vi "Open Front Panel.vi"(6 "Custom Size":cluster{"Height":i16, "Width":i16}, 8 "error in (no error)":errorcluster, 9 "Custom Position":cluster{"Top":i16, "Left":i16}, 10 "Position":T1, 11 "MediatorBusMonitor in":refnum<class "MediatorBusMonitor.lvclass">) -> (0 "error out":errorcluster, 3 "MediatorBusMonitor out":refnum<class "MediatorBusMonitor.lvclass">)   [LabVIEW 2017, in "Mediator.lvlib" / "MediatorBusMonitor.lvclass"]
doc: "<License>\nCopyright © 2017 Composed Systems, LLC | All rights reserved\nwww.composed.io\n\nAuthor: Ethan Stern <ethan.stern@composed.io>\n\nThis software is provided \"AS IS\" WITHOUT WARRANTIES, either express or implied, AND IS FOR EDUCATIONAL PURPOSES ONLY.\n</License>"
uses:
  MediatorBusMonitor.lvclass
  IViewable/IViewable/View Position Enum.ctl
  MediatorBusMonitor.lvclass/MediatorBusMonitor.ctl
  IMediator/IMediatorBusMonitor/MediatorBusMonitor/IMediatorBusMonitor.lvclass
  IViewable/IViewable/IViewable.lvclass
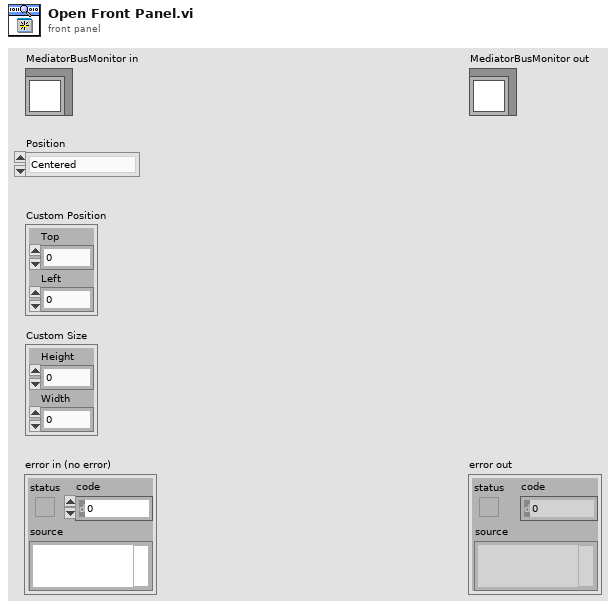
[diagram p1: front panel]
types:
  T1 = typedef "IViewable.lvlib/IViewable.lvclass/View Position Enum.ctl" = enum16{"Centered", "Maximized", "Minimized", "Custom", "Unchanged"}
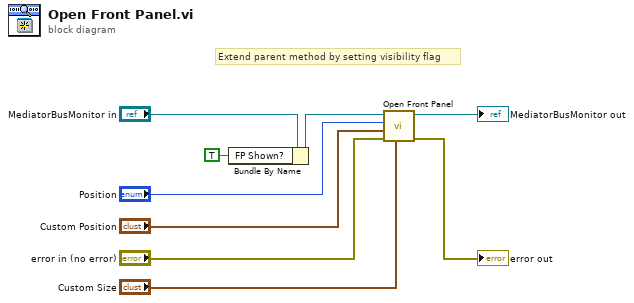
[diagram p0: block diagram]
diagram:
  # "Extend parent method by setting visibility flag"
  n1 = Bundle By Name(cluster="MediatorBusMonitor in", "FP Shown?"=TRUE) -> (w9:refnum<class "MediatorBusMonitor.lvclass">)
  n2 = call-parent "Open Front Panel.vi"("Custom Window Size"="Custom Size", "error in (no error)"="error in (no error)", "Custom Window Position"="Custom Position", "Position"="Position", "IViewable in"=w9) -> ("error out"=→"error out":errorcluster, "IViewable out"=→"MediatorBusMonitor out":refnum<class "MediatorBusMonitor.lvclass">)  [unwired: 5 in]
